vi "subVIweek7pt2.vi"(9 "Length":dbl, 10 "Resistivity":dbl, 11 "Numeric in":dbl) -> (3 "Numeric out":dbl)   [LabVIEW 2016]
uses:
  <vilib>/express/express arith-compare/Formula/XNode/ExpressFormulaBlockNode.xnode
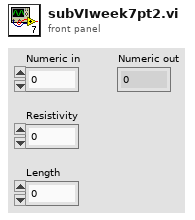
[diagram p1: front panel]
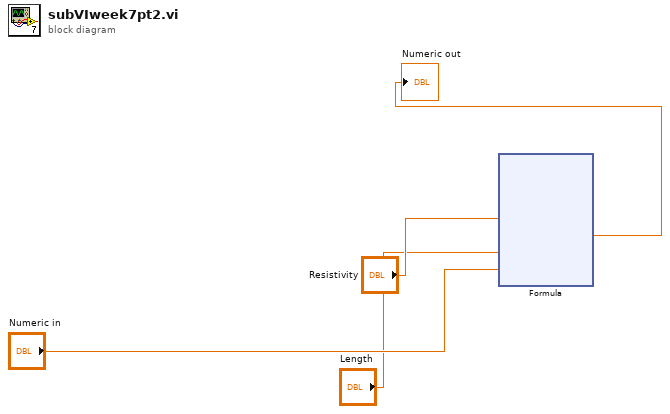
[diagram p0: block diagram]
diagram:
  n1 = xnode "Formula"("X1"="Resistivity", "X2"="Length", "X3"="Numeric in") -> ("Result"=→"Numeric out":dbl)  [unwired: 1 in, 1 out]
